vi "Test1588.vi"() -> ()   [LabVIEW 2014]
uses:
  <instrlib>/niSync/niSync.llb/niSync Initialize (IVI).vi
panel:
  out "time stamp":timestamp
  in  "1588 time":T1
  out "error out 2":errorcluster
  out "error out":errorcluster
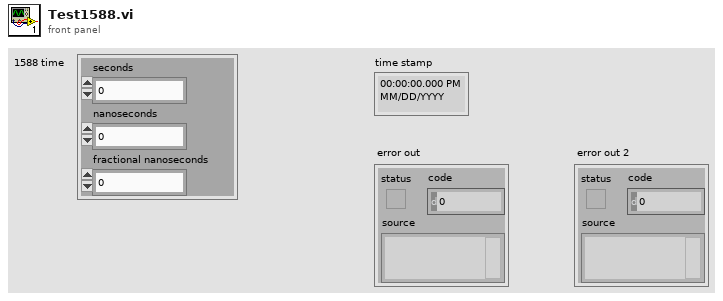
[diagram p1: front panel]
types:
  T1 = cluster{"seconds":u32, "nanoseconds":u32, "fractional nanoseconds ":u16}
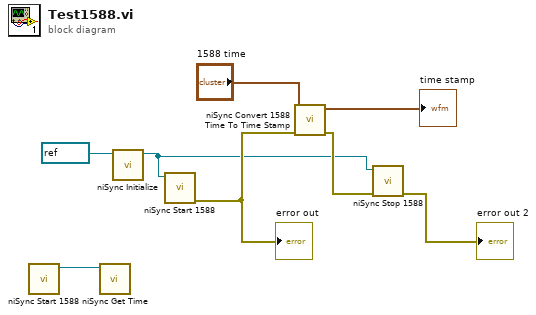
[diagram p0: block diagram]
diagram:
  n1 = call <instrlib>:"niSync Start 1588.vi"() -> ("instrument handle out"=w1:refnum<k15>)  [unwired: 10 in, 1 out]
  n2 = call <instrlib>:"niSync Get Time.vi"("instrument handle"=w1) -> ()  [unwired: 6 in, 3 out]
  n3 = call-poly <instrlib>:"niSync Initialize.vi"("resource name"=refnum<k15> "ptp") -> ("instrument handle out"=w2:refnum<k15>)  [unwired: 9 in, 1 out]
  n4 = call <instrlib>:"niSync Start 1588.vi"("instrument handle"=w2) -> ("error out"=w7:errorcluster)  [unwired: 9 in, 1 out]
  "error out" <- w7
  n5 = call <instrlib>:"niSync Convert 1588 Time To Time Stamp.vi"("error in (no error)"=w7, "1588 time"="1588 time") -> ("error out"=w6:errorcluster, "time stamp"=→"time stamp":timestamp)  [unwired: 8 in]
  n6 = call <instrlib>:"niSync Stop 1588.vi"("error in (no error)"=w6, "instrument handle"=w2) -> ("error out"=→"error out 2":errorcluster)  [unwired: 8 in, 1 out]
